vi "Setup.vi"(5 "Protocol selection\n(appended)":T1 {"Mode" items=["Modbus-1", "3"]}, 7 "protocol selection ref":refnum<vi>, 8 "error in (no error)":errorcluster, 9 "search":bool, 10 "Comm master cluster in":T4={"Main event var"=refnum, "VIRef"=refnum, "Data path"=path "", "Reads"=0, "total number of UUT"=0, "FF refnum"={"Handle1"=0, "Handle2"=0}, "FF device id list"=[], "MODBUS resource name"="", "MODBUS Serial Parameters"={"Mode"=enum."RTU", "Default Slave Address"=0, "MODBUS timeout"=0, "Baud Rate"=0, "Parity"=0, "Flow Control"=0}, "Profibus resource name"="", "Profibus Communication ref.:"=0, "HART resource name"="", "HART long addresses (array)"=[], "Comm relay session"="", "Comm UI event"=refnum, "Write Interval (s)"=5.0, "DMM_QUEUE"=refnum, "POWER_QUEUE"=refnum, "\nTHERM_QUEUE"=refnum, "\nCOMM_QUEUE"=refnum, "TIMING_QUEUE"=refnum, "MAIN_QUEUE"=refnum, "Log path"=path ""} {"Write Interval (s)" min=0.1 max=1000.0 step=0.1}, 11 "MODBUS in":refnum<class "MODBUS.lvclass">) -> (0 "error out":errorcluster, 3 "MODBUS out":refnum<class "MODBUS.lvclass">)   [LabVIEW 2016, in "MODBUS.lvclass"]
uses:
  MODBUS.lvclass
  MASTER_OPC.ctl
  Typedef/event var.ctl
  Typedef/Comm ui action type.ctl
  Typedef/Comm_State_enum.ctl
  Typedef/state var.ctl
  Typedef/Array_of_Comm_mode_and_address_types.ctl
  Typedef/Comm_mode_and_address_type.ctl
  Typedef/Comm_mode_type_combo.ctl
  Typedef/Protocol_enum_type.ctl
  MODBUS.lvclass/MODBUS.ctl
  Protocol Class/Protocol.lvclass
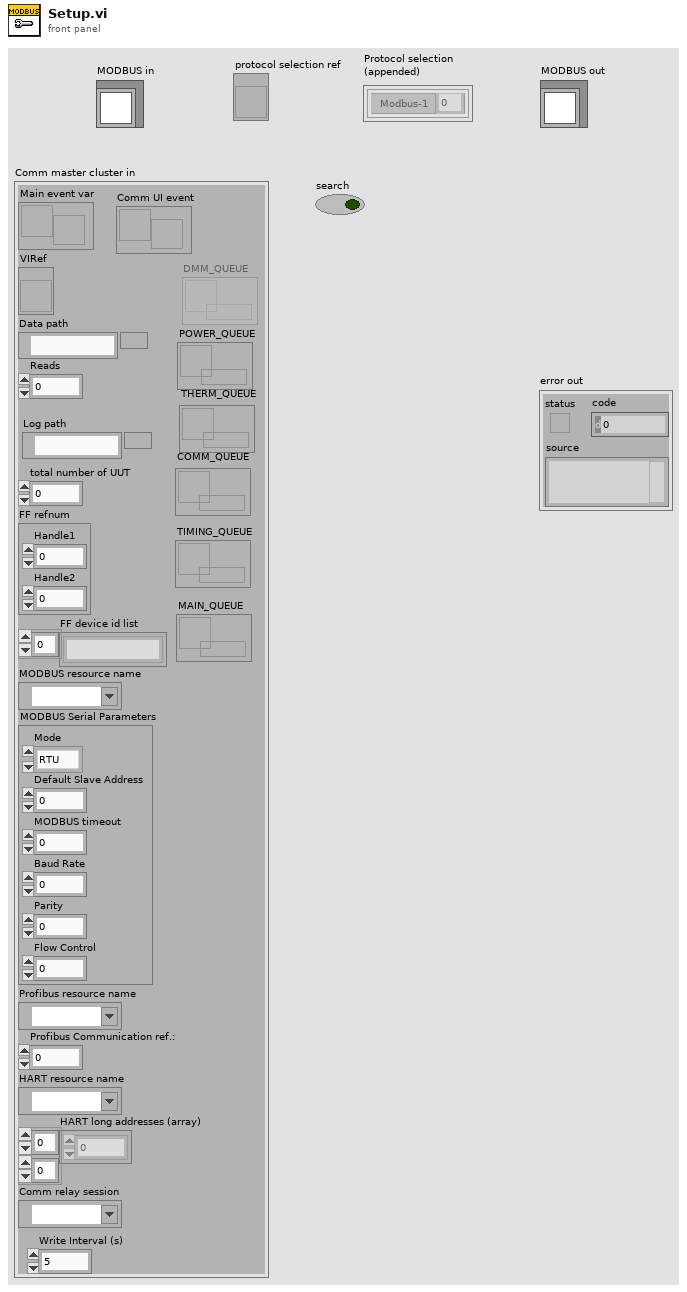
[diagram p1: front panel]
types:
  T1 = typedef "Array_of_Comm_mode_and_address_types.ctl" = T2[]
  T2 = typedef "Comm_mode_and_address_type.ctl" = cluster{"address":i32, "Mode":T3}
  T3 = typedef "Comm_mode_type_combo.ctl" = u16
  T4 = typedef "MASTER_OPC.ctl" = cluster{"Main event var":refnum<user-event>, "VIRef":refnum<vi>, "Data path":path, "Reads":i32, "total number of UUT":i32, "FF refnum":cluster{"Handle1":u32, "Handle2":u32}, "FF device id list":string[], "MODBUS resource name":refnum<visa-resource-name>, "MODBUS Serial Parameters":cluster{"Mode":enum16{"RTU", "ASCII"}, "Default Slave Address":u8, "MODBUS timeout":u32, "Baud Rate":u32, "Parity":u16, "Flow Control":u16}, "Profibus resource name":refnum<visa-resource-name>, "Profibus Communication ref.:":u8, "HART resource name":refnum<visa-resource-name>, "HART long addresses (array)":u8[][], "Comm relay session":refnum<k15>, "Comm UI event":refnum<user-event>, "Write Interval (s)":dbl, "DMM_QUEUE":refnum<queue>, "POWER_QUEUE":refnum<queue>, "\nTHERM_QUEUE":refnum<queue>, "\nCOMM_QUEUE":refnum<queue>, "TIMING_QUEUE":refnum<queue>, "MAIN_QUEUE":refnum<queue>, "Log path":path}
  T5 = typedef "Protocol_enum_type.ctl" = enum16{"None", "MODBUS", "HART", "Fieldbus", "Profibus DP", "Profibus PA", "DeviceNET", "USB"}
  T6 = enum16{"Connect whole bus", "Connect individual UUTs", "Connect none"}
  T7 = cluster{"Device address":i32, "Switch index":i32}
  T8 = typedef "MODBUS parameters type.ctl" = cluster{"Mode":enum16{"RTU", "ASCII"}, "Default Slave Address":u8, "MODBUS timeout":u32, "Baud Rate":u32, "Parity":u16, "Flow Control":u16}
  T9 = cluster{"Device address":i32, "Switch index":i32}[]
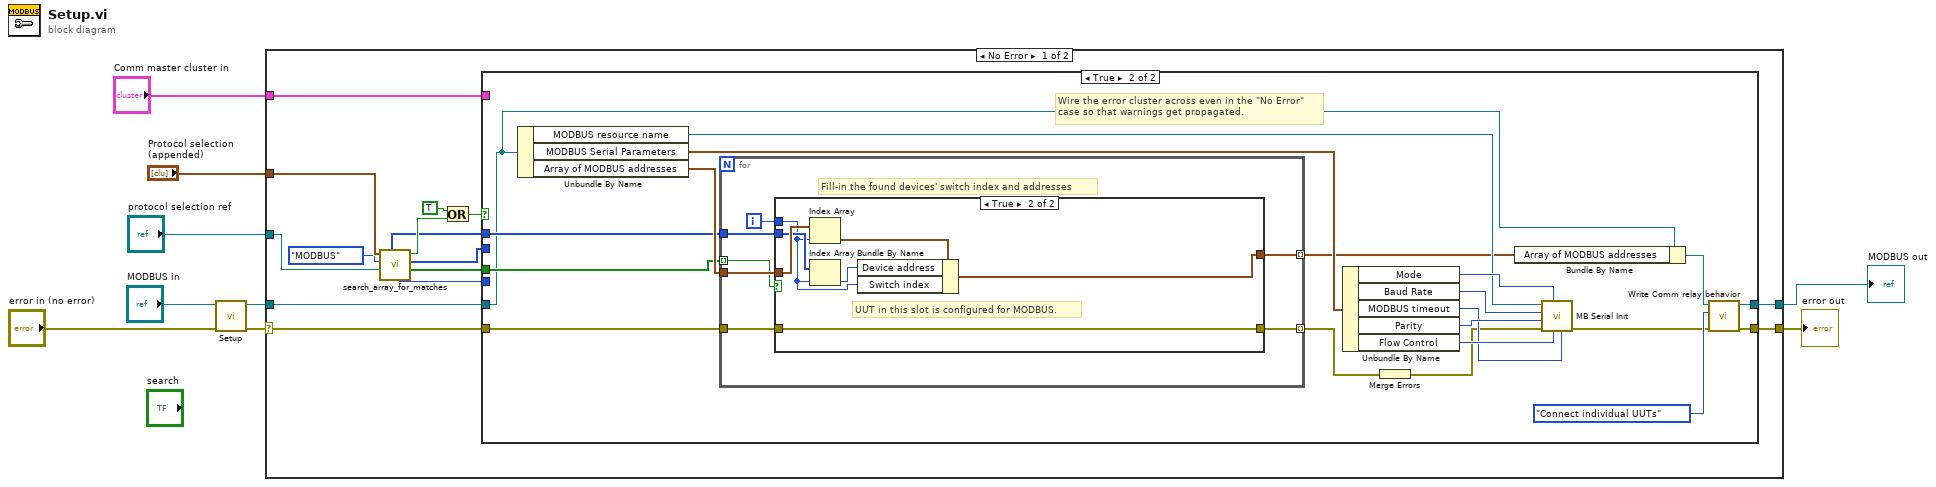
[diagram p0: block diagram]
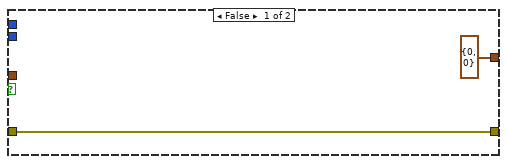
[diagram p3: hidden frame]
diagram:
  n1 = call-parent "Setup.vi"("error in (no error)"="error in (no error)", "Protocol in"="MODBUS in") -> ("error out"=w7:errorcluster, "Protocol out"=w5:refnum<class "MODBUS.lvclass">)  [unwired: 8 in]
  n2 = case shown="No Error" w7 {
    selector: w7 -> [w24 w63]
    tunnel: [w23 w63] -> w6
    tunnel: w5 -> [w22 w64]
    tunnel: [w12 w64] -> w4
    tunnel: "Comm master cluster in" -> [w15 _]
    tunnel: "Protocol selection\n(appended)" -> [w21 _]
    tunnel: "protocol selection ref" -> [w20 _]
    frame No Error {
      n3 = call "search_array_for_matches.vi"("protocol selection ref"=w20, "Protocol enum"=Protocol_enum_type."MODBUS", "appended array"=w21) -> ("Array of exists"=w17:bool[], "array of indexes"=w13:i32[], "exists?"=w18:bool, "Switch Row"=w14:i32, "all addresses"=w16:i32[])  [unwired: 3 in, 1 out]
      n4 = Or(x=TRUE, y=w18) -> (x .or. y?=w11:bool)
      n5 = case shown="True" w11 {
        tunnel: w24 -> [w26 w27]
        tunnel: [w26 w28] -> w23
        tunnel: w22 -> [w25 w33]
        tunnel: w16 -> [_ w36]
        tunnel: w17 -> [_ w37]
        tunnel: w15 -> [_ _]
        tunnel: w14 -> [_ _]
        tunnel: w13 -> [_ _]
        tunnel: [w25 w30] -> w12
        frame False {
        }
        frame True {
          # "Wire the error cluster across even in the \"No Error\"\ncase so that warnings get propagated."
          n6 = Unbundle By Name(w33) -> ("MODBUS resource name"=w41:refnum<visa-resource-name>, "MODBUS Serial Parameters"=w40:T8, "Array of MODBUS addresses"=w39:T9)
          n7 = for {
            tunnel: w39 -> [w53]
            tunnel: [w52] -> w34 mode=indexing
            tunnel: w27 -> [w51]
            tunnel: [w50] -> w38 mode=indexing
            tunnel: w37 -> [w49] mode=indexing
            tunnel: w36 -> [w47]
            i -> [w48]
            # "Fill-in the found devices' switch index and addresses"
            n8 = case shown="True" w49 {
              tunnel: w53 -> [_ w62]
              tunnel: w47 -> [_ w61]
              tunnel: [T7 {"Device address"=0, "Switch index"=0} ("Hart address") w56] -> w52
              tunnel: w51 -> [w55 w58]
              tunnel: [w55 w58] -> w50
              tunnel: w48 -> [_ w59]
              frame False {
              }
              frame True {
                # "UUT in this slot is configured for MODBUS."
                n9 = Index Array(array=w62, index=w59) -> (element=w60:T7)
                n10 = Index Array(array=w61, index=w59) -> (element=w57:i32)
                n11 = Bundle By Name(cluster=w60, "Device address"=w57, "Switch index"=w59) -> (w56:T7)
              }
            }
          }
          n12 = Unbundle By Name(w40) -> ("Mode"=w46:enum16{"RTU", "ASCII"}, "Baud Rate"=w45:u32, "MODBUS timeout"=w42:u32, "Parity"=w44:u16, "Flow Control"=w43:u16)
          n13 = Merge Errors(w38) -> (w35:errorcluster)
          n14 = Bundle By Name(cluster=w33, "Array of MODBUS addresses"=w34) -> (w32:refnum<class "MODBUS.lvclass">)
          n15 = call "MB Serial Init.vi"("Timeout"=w42, "Flow Control"=w43, "Mode"=w46, "error in (no error)"=w35, "Parity"=w44, "Baud Rate"=w45, "VISA resource name"=w41) -> ("error out"=w29:errorcluster)  [unwired: 4 out]
          n16 = call-dynamic "Write Comm relay behavior.vi"("error in (no error)"=w29, "Comm relay behavior"=T6."Connect individual UUTs", "Protocol in"=w32) -> ("error out"=w28:errorcluster, "Protocol out"=w30:refnum<class "MODBUS.lvclass">)  [unwired: 7 in]
        }
      }
    }
    frame Error {
    }
  }
  "error out" <- w6
  "MODBUS out" <- w4
